vi "TREE_LIST_convert a tree to a list.vi"(8 "error in (no error)":errorcluster, 9 "directory file names":string[](array[string]), 10 "selectrd item (path)":path) -> (0 "error out":errorcluster, 2 "File info out":string[][](array[string]))   [LabVIEW 2011]
uses:
  <userlib>/_OpenG.lib/file/file.llb/Strip Path__ogtk.vi
  <userlib>/_OpenG.lib/file/file.llb/Build Path__ogtk.vi
  <userlib>/_OpenG.lib/file/file.llb/File Exists - Scalar__ogtk.vi
  <userlib>/_OpenG.lib/file/file.llb/Strip Path Extension__ogtk.vi
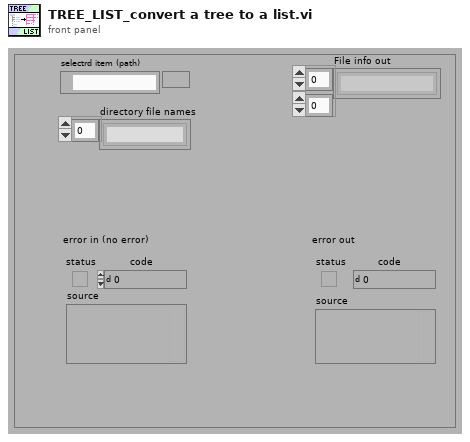
[diagram p1: front panel]
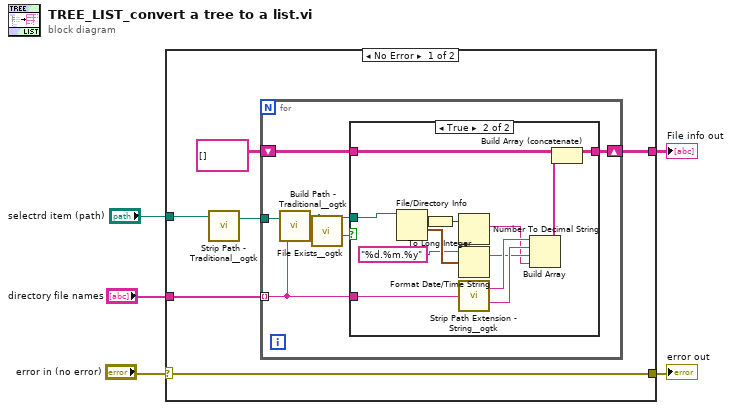
[diagram p0: block diagram]
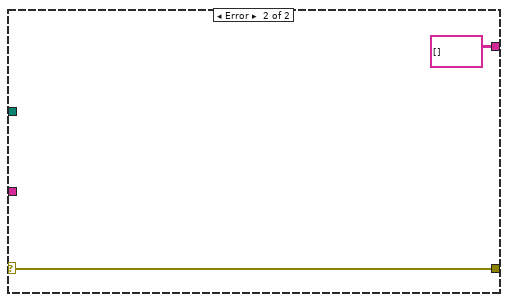
[diagram p3: hidden frame]
diagram:
  n1 = case shown="No Error" "error in (no error)" {
    selector: "error in (no error)" -> [w6 w32]
    tunnel: [w11 string[][] []] -> w5
    tunnel: "selectrd item (path)" -> [w8 _]
    tunnel: "directory file names" -> [w7 _]
    tunnel: [w6 w32] -> w1
    frame No Error {
      n2 = call-poly <userlib>:"Strip Path - Traditional__ogtk.vi"("path"=w8) -> ("stripped path"=w9:path)  [unwired: 1 out]
      n3 = for {
        tunnel: w7 -> [w16] mode=indexing
        tunnel: w9 -> [w17]
        shift-right: [w12] -> w11
        shift-left: string[][] [] -> [w13]
        n4 = call-poly <userlib>:"Build Path - Traditional__ogtk.vi"("name or relative path"=w16, "base path"=w17) -> ("appended path"=w15:path)
        n5 = call-poly <userlib>:"File Exists__ogtk.vi"("file path"=w15) -> ("exists"=w14:bool)  [unwired: 6 in, 1 out]
        n6 = case shown="True" w14 {
          tunnel: w16 -> [_ w28]
          tunnel: w15 -> [_ w23]
          tunnel: w13 -> [w18 w21]
          tunnel: [w18 w22] -> w12
          frame False {
          }
          frame True {
            n7 = File/Directory Info(path=w23) -> (size=w19:i64, last mod=w30:timestamp)  [unwired: 1 in, 5 out]
            n8 = To Long Integer(number=w19) -> (32bit integer=w31:i32)
            n9 = Number To Decimal String(number=w31) -> (decimal integer string=w24:string)  [unwired: 1 in]
            n10 = Format Date/Time String(time format string (%c)="%d.%m.%y", seconds (now)=w30) -> (date/time string=w25:string)  [unwired: 1 in]
            n11 = call-poly <userlib>:"Strip Path Extension - String__ogtk.vi"("path"=w28) -> ("root"=w27:string, "extension"=w26:string)
            n12 = Build Array(w27, w26, w25, w24) -> (w20:string[])
            n13 = Build Array (concatenate)(w21, w20) -> (w22:string[][])
          }
        }
      }
    }
    frame Error {
    }
  }
  "File info out" <- w5
  "error out" <- w1
